vi "Draw.vi"(7 "menu in":refnum<class "menu.lvclass">, 8 "error in (no error)":errorcluster, 11 "overlay in":refnum<class "overlay.lvclass">) -> (0 "error out":errorcluster, 3 "overlay out":refnum<class "overlay.lvclass">)   [LabVIEW 2009, in "overlay.lvclass"]
uses:
  overlay.lvclass
  Menu/menu.lvclass
  overlay.lvclass/overlay.ctl
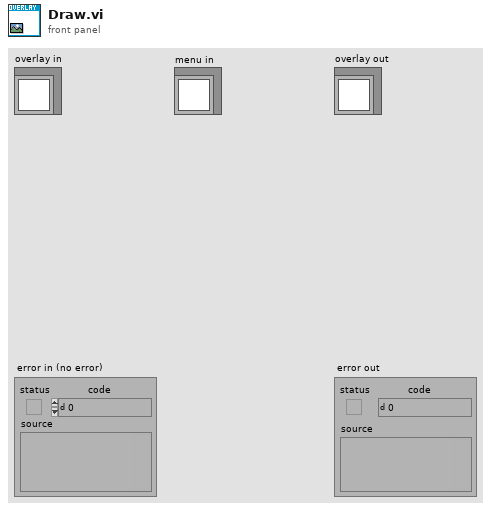
[diagram p1: front panel]
types:
  T1 = cluster{"left":i16, "top":i16, "right":i16, "bottom":i16}
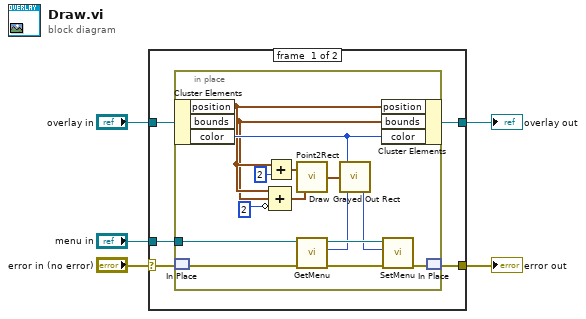
[diagram p0: block diagram]
diagram:
  n1 = case shown="No Error" "error in (no error)" {
    selector: "error in (no error)" -> [w8 w27]
    tunnel: [w7 w27] -> w2
    tunnel: [w6 w26] -> w4
    tunnel: "overlay in" -> [w10 w26]
    tunnel: "menu in" -> [w9 _]
    frame #0 {
      n2 = in-place {
        in-place-border: w9 -> [w20]
        n3 = in-place-cluster #1(w10) -> ("position"=w14:cluster{"left":u32, "top":u32}, "bounds"=w13:cluster{"width":u32, "height":u32}, "color"=w24:u32)
        n4 = in-place-match #2(w8) -> (w23:errorcluster)
        n5 = Add(x=w14, y=i16 2 ("oval width")) -> (x+y=w16:cluster{"left":u32, "top":u32})
        n6 = Compound Arithmetic op=ADD(w14, w13, invert i16 2 ("oval width")) -> (w11:cluster{u32, u32})
        n7 = call <vilib>:"Point2Rect.vi"("point b"=w11, "point a"=w16) -> ("rect"=w25:T1)
        n8 = call "GetMenu.vi"("error in (no error)"=w23, "menu in"=w20) -> ("error out"=w19:errorcluster, "menu"=w18:picture, "menu out"=w21:refnum<class "menu.lvclass">)  [unwired: 7 in]
        n9 = call <vilib>:"Draw Grayed Out Rect.vi"("color(black)"=w24, "rect"=w25, "picture"=w18) -> ("new picture"=w17:picture)  [unwired: 2 in]
        n10 = in-place-cluster #1("position"=w14, "bounds"=w13, "color"=w24) -> (w6:refnum<class "overlay.lvclass">)
        n11 = call "SetMenu.vi"("error in (no error)"=w19, "menu"=w17, "menu in"=w21) -> ("error out"=w22:errorcluster)  [unwired: 7 in, 1 out]
        n12 = in-place-match #2(w22) -> (w7:errorcluster)
      }
    }
    frame #1 {
    }
  }
  "overlay out" <- w4
  "error out" <- w2
